vi "_RT_Pub_WaitCmd.vi"(9 "milliseconds to wait":u32, 10 "error in (no error)":errorcluster) -> (2 "error out":errorcluster)   [LabVIEW 2018]
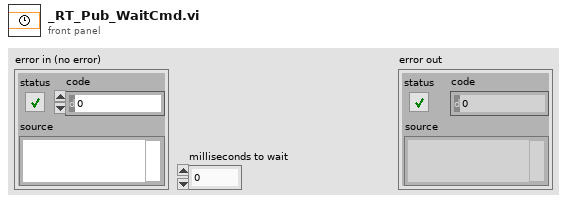
[diagram p1: front panel]
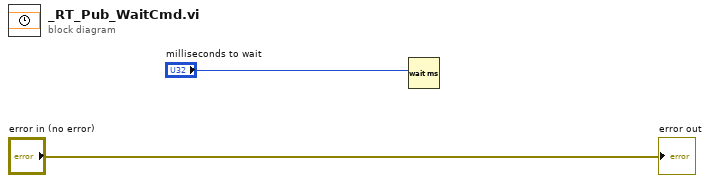
[diagram p0: block diagram]
diagram:
  n1 = Wait (ms)(milliseconds to wait="milliseconds to wait") -> ()  [unwired: 1 out]
  "error out" <- "error in (no error)"
